vi "JAS-Color Sensor V3 Color Match FGV.vi"(9 "UpdateIndex":i32 min=0, 10 "ColorMatchFGV-Cmd":T1, 11 "Color Match":T2) -> (2 "LastIndex":i32, 3 "All Match Colors":T2[](array[typedef]))   [LabVIEW 2019]
uses:
  <vilib>/Rock Robotics/WPI/ThirdParty/REV Robotics/Color SensorV3/Typedef/Color Sensor V3 Color Match.ctl
  JAS-ColorMatch-FGV-Cmd.ctl
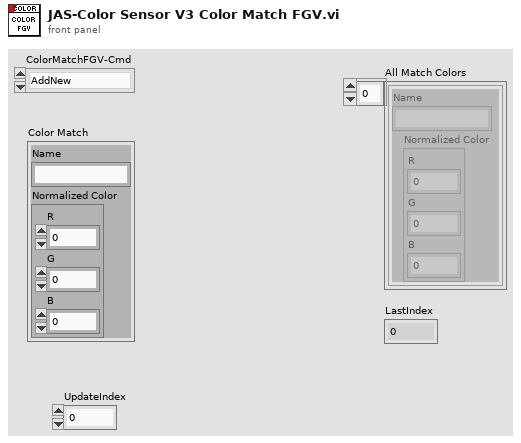
[diagram p1: front panel]
types:
  T1 = typedef "JAS-ColorMatch-FGV-Cmd.ctl" = enum16{"AddNew", "Update", "Read"}
  T2 = typedef "Color Sensor V3 Color Match.ctl" = cluster{"Name":string, "Normalized Color":cluster{"R":dbl, "G":dbl, "B":dbl}}
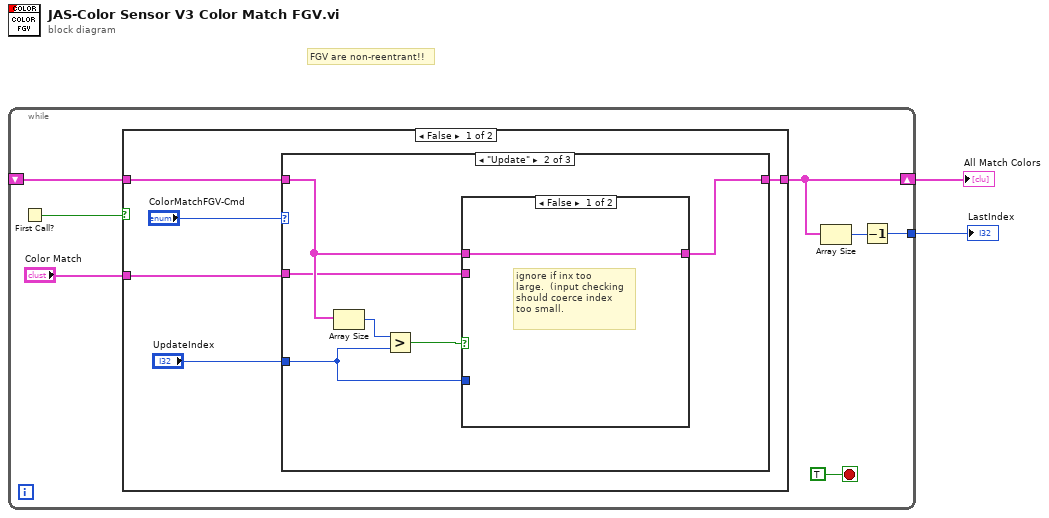
[diagram p0: block diagram]
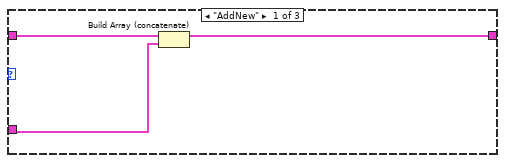
[diagram p2: hidden frame]
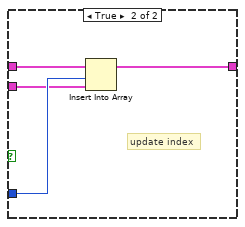
[diagram p3: hidden frame]
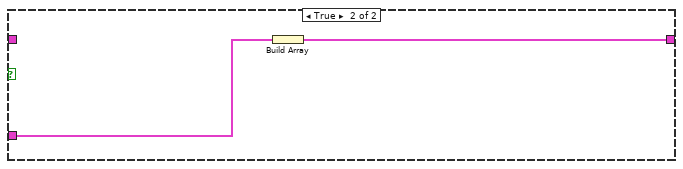
[diagram p5: hidden frame]
diagram:
  # "FGV are non-reentrant!!"
  n1 = while {
    shift-right: [w5] -> w2
    shift-left: _ -> [w7]
    tunnel: [w3] -> w1
    stop <- TRUE stop-if-true
    n2 = First Call?() -> (First Call?: T/F=w8:bool)
    n3 = case shown="False" w8 {
      tunnel: "Color Match" -> [w14 w31]
      tunnel: [w12 w30] -> w5
      tunnel: w7 -> [w13 _]
      frame False {
        n4 = case shown="\"Update\"" "ColorMatchFGV-Cmd" {
          tunnel: w14 -> [w17 w18 _]
          tunnel: w13 -> [w16 w21 w29]
          tunnel: [w15 w20 w29] -> w12
          tunnel: "UpdateIndex" -> [_ w19 _]
          frame "AddNew" {
            n5 = Build Array (concatenate)(w16, w17) -> (w15:T2[])
          }
          frame "Update" {
            n6 = Array Size(array=w21) -> (size(s)=w23:i32)
            n7 = Greater?(x=w23, y=w19) -> (0:w22:bool)
            n8 = case shown="False" w22 {
              tunnel: w21 -> [w24 w28]
              tunnel: [w24 w27] -> w20
              tunnel: w19 -> [_ w26]
              tunnel: w18 -> [_ w25]
              frame False {
                # "ignore if inx too\nlarge.  (input checking\nshould coerce index\ntoo small."
              }
              frame True {
                # "update index"
                n9 = Insert Into Array(array=w28, index=w26, new element=w25) -> (w27:T2[])
              }
            }
          }
          frame "Read" {
          }
        }
      }
      frame True {
        n10 = Build Array(w31) -> (w30:T2[])
      }
    }
    n11 = Array Size(array=w5) -> (size(s)=w4:i32)
    n12 = Decrement(x=w4) -> (x-1=w3:i32)
  }
  "All Match Colors" <- w2
  "LastIndex" <- w1
